vi "Update-index.vi"(8 "error in (no error)":errorcluster, 9 "Image ok?":bool=TRUE, 10 "Index in":i32) -> (0 "error out":errorcluster, 2 "Index":i32)   [LabVIEW 2013, in "CameraVision.lvlib" / "CV-Acquisition.lvclass"]
uses:
  CV-Acquisition.lvclass
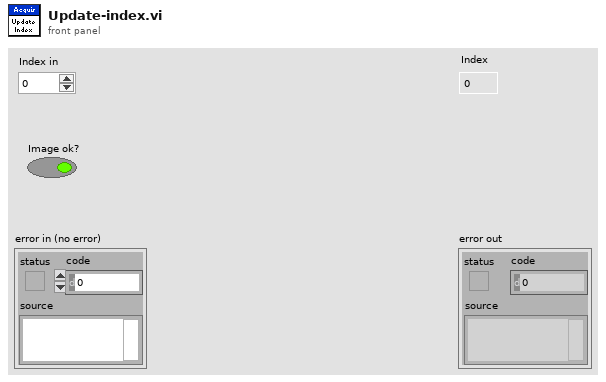
[diagram p1: front panel]
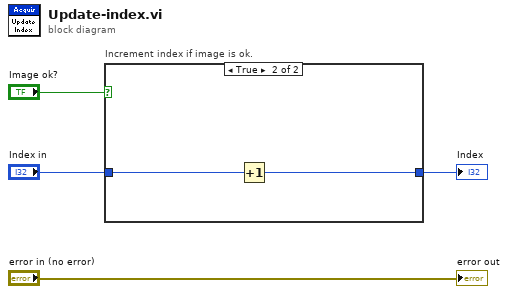
[diagram p0: block diagram]
diagram:
  n1 = case "Increment index if image is ok." shown="True" "Image ok?" {
    tunnel: "Index in" -> [w5 w7]
    tunnel: [w5 w6] -> w1
    frame False {
    }
    frame True {
      n2 = Increment(x=w7) -> (x+1=w6:i32)
    }
  }
  "Index" <- w1
  "error out" <- "error in (no error)"
